vi "CallAddresses.vi"(7 "Module Cluster In":T2, 8 "error in (no error)":errorcluster, 10 "Local Ip":string) -> (0 "error out":errorcluster, 1 "Response Array":T1[](array[typedef]), 5 "Module Cluster Out":T2)   [LabVIEW 2020, in "Controller.lvlib"]
uses:
  Controller.lvlib
  Public Controls/Module Data Cluster.ctl
  Public Controls/Config.ctl
  Public Controls/IP Address Response Type Def.ctl
  Public Controls/IP Stats.ctl
  UI/UI.lvlib
panel:
  out "Array":string[](array[string])
  out "array":string[](array[string])
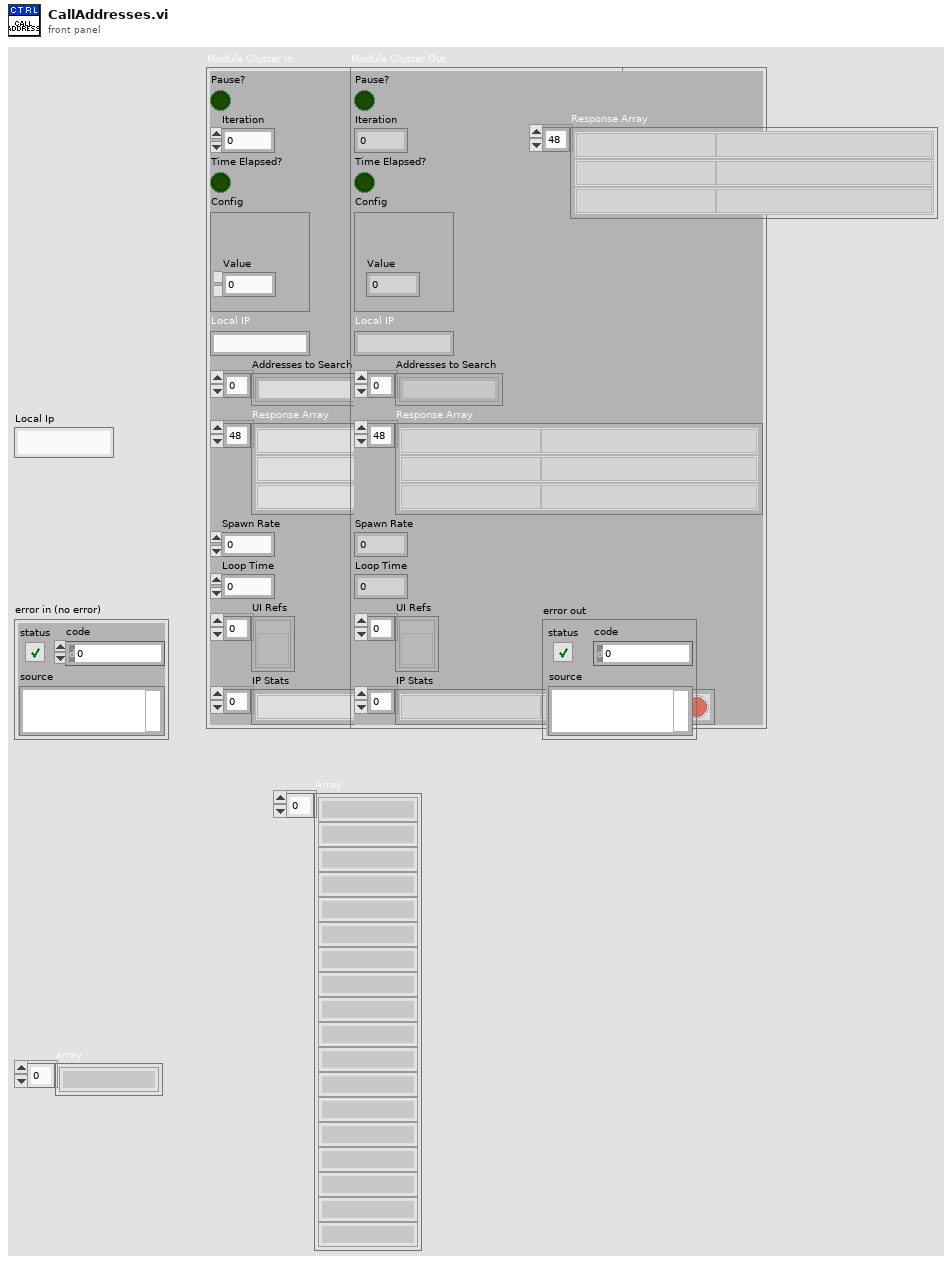
[diagram p1: front panel]
types:
  T1 = typedef "UI.lvlib/IP Address Response Type Def.ctl" = cluster{"Address":string, "Response":string}
  T2 = typedef "Controller.lvlib/Module Data Cluster.ctl" = cluster{"Pause?":bool, "Iteration":i32, "Time Elapsed?":bool, "Config":T3, "Local IP":string, "Addresses to Search":string[], "Response Array":T1[], "Spawn Rate":i32, "Loop Time":u32, "UI Refs":refnum<vi>[], "IP Stats":T4[]}
  T3 = typedef "Controller.lvlib/Config.ctl" = cluster{"Value":dbl}
  T4 = typedef "UI.lvlib/IP Stats.ctl" = cluster{"Address":string, "Average Response Time":i32, "Loss %":i32, "Min Response Time":i32, "Max Response Time":i32, "Boolean":bool}
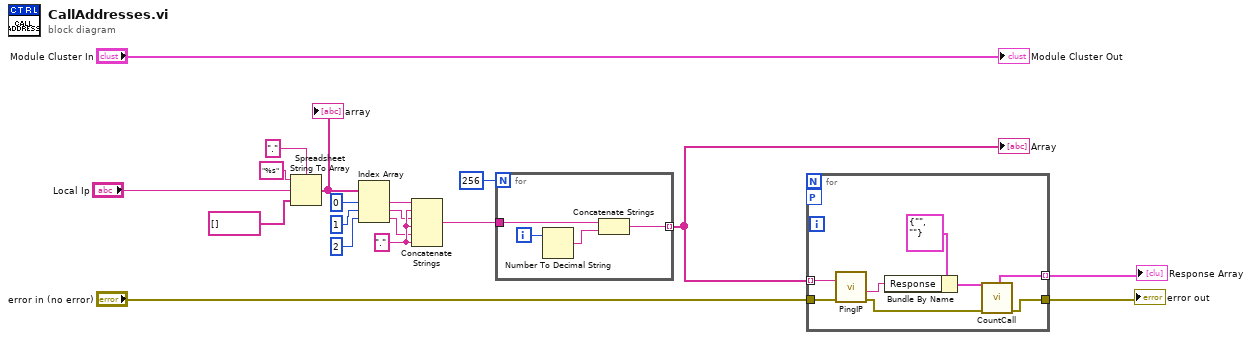
[diagram p0: block diagram]
diagram:
  w12 = "." ("delimiter (Tab)")
  n1 = Spreadsheet String To Array(delimiter (Tab)=".", format string="%s" ("spreadsheet string"), spreadsheet string="Local Ip", array type (2D Dbl)=string[] []) -> (array=w16:string[])
  "array" <- w16
  n2 = Index Array(array=w16, index #1=0 ("index"), index #2=1 ("index"), index #3=2 ("index")) -> (element #1=w11:string, element #2=w10:string, element #3=w9:string)
  n3 = Concatenate Strings(w11, w12, w10, w12, w9, w12) -> (w7:string)
  n4 = for {
    N: 256 -> [_]
    tunnel: w7 -> [w22]
    tunnel: [w23] -> w2 mode=indexing
    i -> [w20]
    n5 = Number To Decimal String(number=w20) -> (decimal integer string=w21:string)  [unwired: 1 in]
    n6 = Concatenate Strings(w22, w21) -> (w23:string)
  }
  "Array" <- w2
  n7 = for {
    tunnel: w2 -> [w30] mode=indexing
    tunnel: [w25] -> w5
    tunnel: "error in (no error)" -> [w29]
    tunnel: [w24] -> w4 mode=indexing
    workers-P: _ -> [_]
    n8 = call "PingIP.vi"("error in (no error)"=w29, "IP Address"=w30) -> ("error out"=w26:errorcluster, "Ping Response"=w27:string)  [unwired: 8 in]
    n9 = Bundle By Name(cluster=T1 {"Address"="", "Response"=""} ("Address Response"), "Response"=w27) -> (w24:T1)
    n10 = call "CountCall.vi"("error in (no error)"=w26) -> ("error out"=w25:errorcluster)  [unwired: 10 in]
  }
  "error out" <- w5
  "Response Array" <- w4
  "Module Cluster Out" <- "Module Cluster In"
